vi "dfd_Merge FLP and FXP Analysis Outputs (Log-Spaced).vi"(5 "output option":u16(ring) items=["Auto", "Floating-Point Only", "Fixed-Point Only"], 7 "frequency points":dbl[](array[numeric]), 8 "error in FXP":errorcluster, 9 "response FXP":dbl[](array[numeric]) format="%.2f", 10 "error in FLP":errorcluster, 11 "response FLP":dbl[](array[numeric]) format="%.2f") -> (0 "error out":errorcluster, 3 "freq responses":cluster{"bins":dbl[], "response FXP":dbl[]}[](array[cluster]))   [LabVIEW 2017, in "NI_DigFilterLicensed.lvlib"]
uses:
  <vilib>/addons/Digital Filter Design/NI_DigFilterLicensed.lvlib
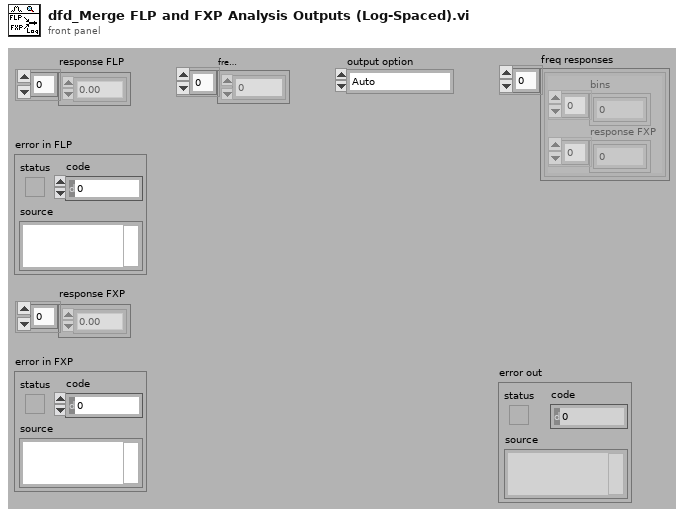
[diagram p1: front panel]
types:
  T1 = cluster{"frequency points":dbl[], "response FLP":dbl[]}
  T2 = cluster{"frequency points":dbl[], "response FXP":dbl[]}
  T3 = cluster{"frequency points":dbl[], "response FXP":dbl[]}[]
  T4 = cluster{"frequency points":dbl[], "response FLP":dbl[]}[]
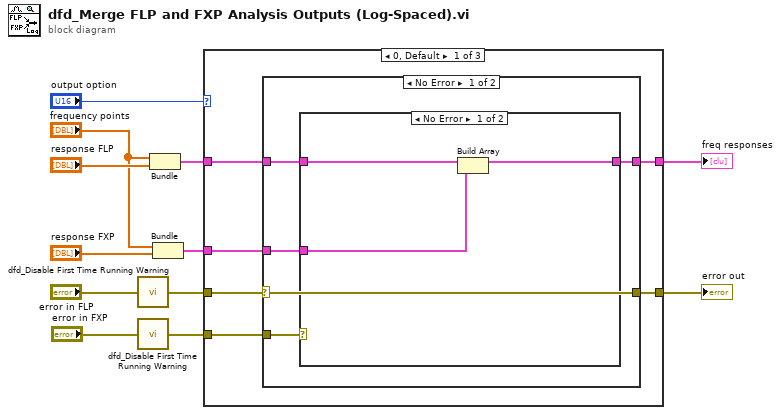
[diagram p0: block diagram]
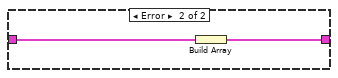
[diagram p2: hidden frame]
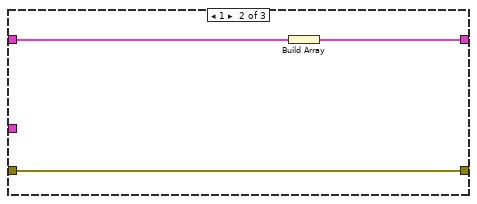
[diagram p4: hidden frame]
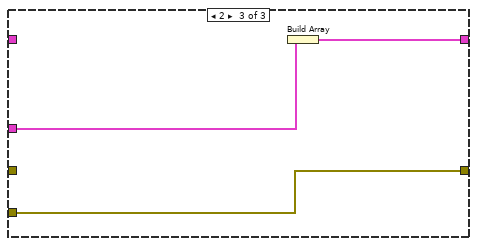
[diagram p5: hidden frame]
diagram:
  n1 = call <vilib>:"dfd_Disable First Time Running Warning.vi"("error in"="error in FLP") -> ("error out"=w5:errorcluster)  [unwired: 1 in]
  n2 = call <vilib>:"dfd_Disable First Time Running Warning.vi"("error in"="error in FXP") -> ("error out"=w3:errorcluster)  [unwired: 1 in]
  n3 = Bundle("frequency points"="frequency points", "response FLP"="response FLP") -> (w8:T1)  [unwired: 1 out]
  n4 = Bundle("frequency points"="frequency points", "response FXP"="response FXP") -> (w6:T2)  [unwired: 1 out]
  n5 = case shown="0, Default" "output option" {
    tunnel: w8 -> [w16 w32 _]
    tunnel: w6 -> [w14 _ w34]
    tunnel: w5 -> [w18 w30 _]
    tunnel: w3 -> [w17 _ w33]
    tunnel: [w15 w31 w35] -> w1
    tunnel: [w13 w30 w33] -> w10
    frame 0, Default {
      n6 = case shown="No Error" w18 {
        selector: w18 -> [w19 w29]
        tunnel: w17 -> [w23 _]
        tunnel: w16 -> [w22 _]
        tunnel: [w21 _] -> w15
        tunnel: w14 -> [w20 _]
        tunnel: [w19 w29] -> w13
        frame No Error {
          n7 = case shown="No Error" w23 {
            tunnel: w22 -> [w26 w28]
            tunnel: [w24 w27] -> w21
            tunnel: w20 -> [w25 _]
            frame No Error {
              n8 = Build Array(w26, w25) -> (w24:T3)
            }
            frame Error {
              n9 = Build Array(w28) -> (w27:T4)
            }
          }
        }
        frame Error {
        }
      }
    }
    frame 1 {
      n10 = Build Array(w32) -> (w31:T4)
    }
    frame 2 {
      n11 = Build Array(w34) -> (w35:T3)
    }
  }
  "error out" <- w10
  "freq responses" <- w1
